vi "Validate number of visits per cave.vi"(11 "Array":i32[](array[numeric])) -> (3 "Invalid?":bool)   [LabVIEW 2019, in "Day 12.lvlib"]
uses:
  Day 12.lvlib
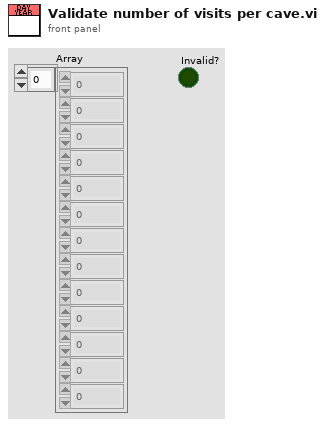
[diagram p1: front panel]
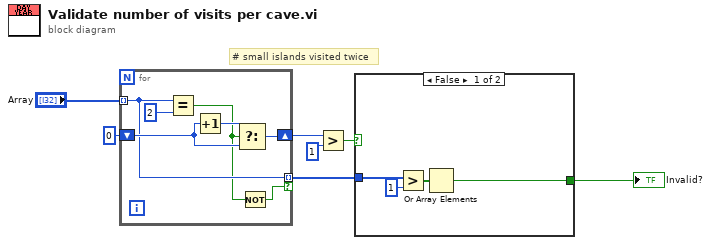
[diagram p0: block diagram]
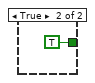
[diagram p2: hidden frame]
diagram:
  # "# small islands visited twice"
  n1 = for {
    tunnel: "Array" -> [w10] mode=indexing
    shift-right: [w13] -> w3
    shift-left: 0 ("y") -> [w12]
    tunnel: [w10] -> w6 mode=indexing if=w9
    n2 = Equal?(x=w10, y=2) -> (x = y?=w8:bool)
    n3 = Increment(x=w12) -> (x+1=w11:i32)
    n4 = Select(t=w11, s=w8, f=w12) -> (s? t:f=w13:i32)
    n5 = Not(x=w8) -> (.not. x?=w9:bool)
  }
  n6 = Greater?(x=w3, y=1) -> (0:w5:bool)
  n7 = case shown="False" w5 {
    tunnel: w6 -> [w16 _]
    tunnel: [w15 TRUE] -> w7
    frame False {
      n8 = Greater?(x=w16, y=1) -> (0:w18:bool[])
      n9 = Or Array Elements(Boolean array=w18) -> (logical OR=w15:bool)
    }
    frame True {
    }
  }
  "Invalid?" <- w7
